vi "CTREPCM_PanelSim_Global.vi"(0 "Menu":T3=enum."delete", 5 "Channel":i32, 7 "Boolean Value":bool, 9 "Numeric Value":dbl format="%#.4f", 11 "error in (no error)":errorcluster, 12 "String Value":string) -> (10 "Value out":T1={"type"="CTREPCM", "device"="", "name"="", "data"={"<init"=FALSE, ">on"=FALSE, "<closed_loop"=FALSE, ">pressure_switch"=FALSE, ">current"=0.0}}, 15 "error out":errorcluster)   [LabVIEW 2019]
doc: "This is used to set and get the last motor output values. This is needed for simulation, since we cannot read these values from the hardware.\n\nThis software is licensed. Open the labview\\readme\\WPI Robotics Library Open Source License.txt file for more information."
uses:
  CTREPCM Update Ops.ctl
  CTREPCM proto.ctl
  CTREPCM Data proto.ctl
panel:
  out "All Values":T1[](array[typedef])
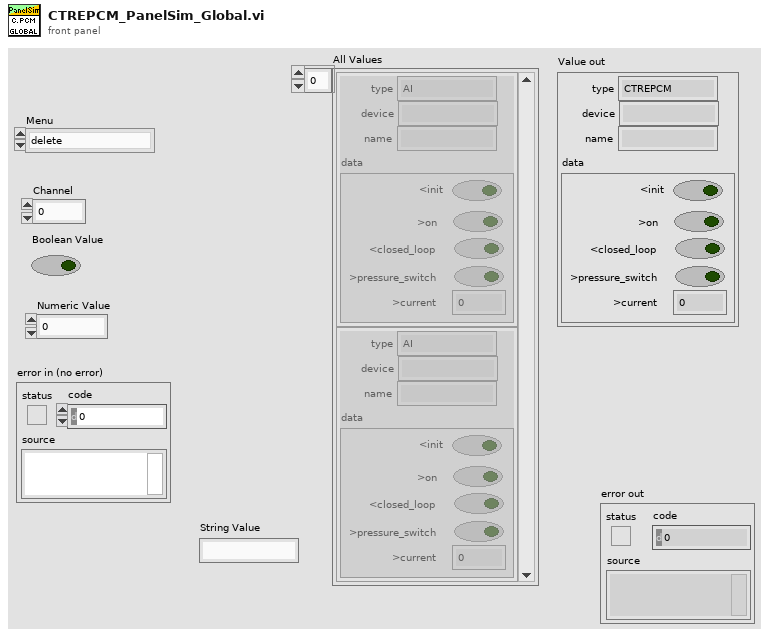
[diagram p1: front panel]
types:
  T1 = typedef "CTREPCM proto.ctl" = cluster{"type":string, "device":string, "name":string, "data":T2}
  T2 = typedef "CTREPCM Data proto.ctl" = cluster{"<init":bool, ">on":bool, "<closed_loop":bool, ">pressure_switch":bool, ">current":dbl}
  T3 = typedef "CTREPCM Update Ops.ctl" = enum16{"get", "delete", "JSON update", "set  name", "transmit initial", "reset", "set init", "set compressor on", "set closed loop", "set pressure switch", "set current"}
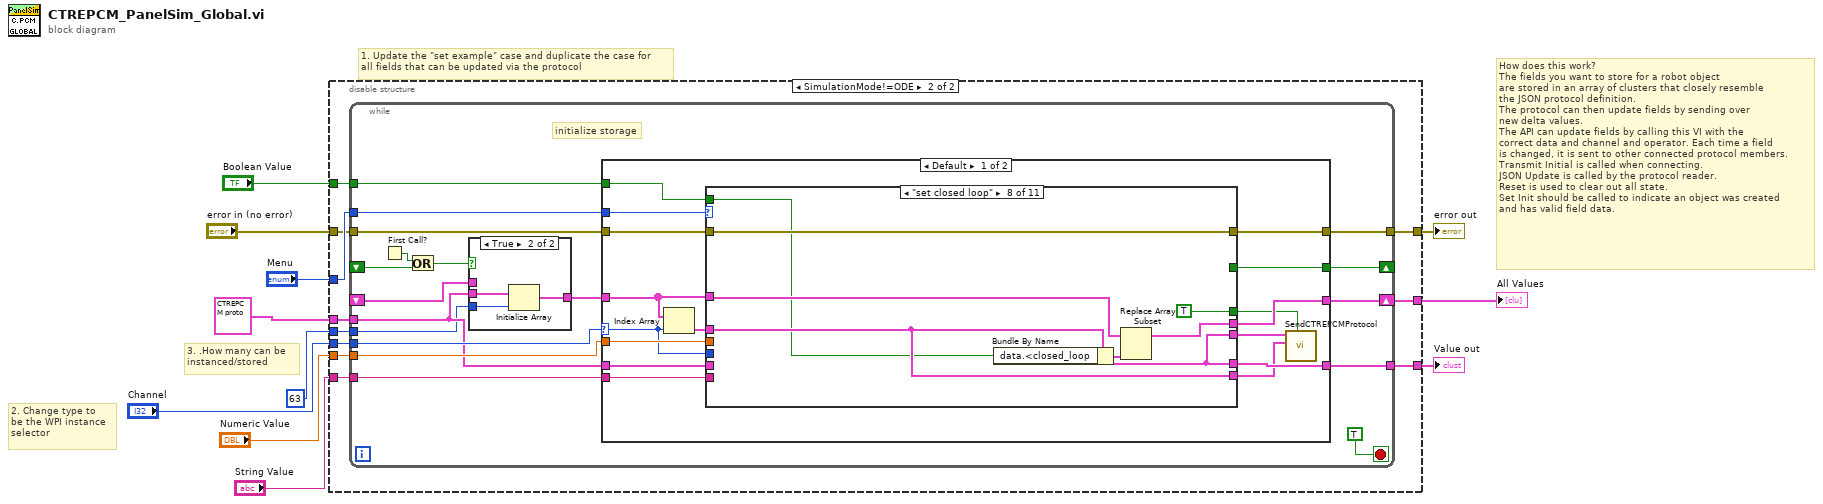
[diagram p0: block diagram]
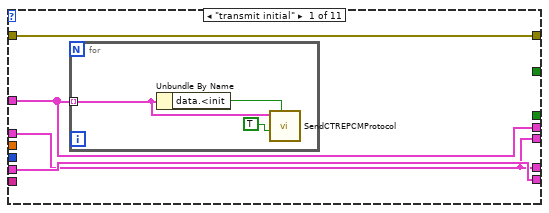
[diagram p3: hidden frame]
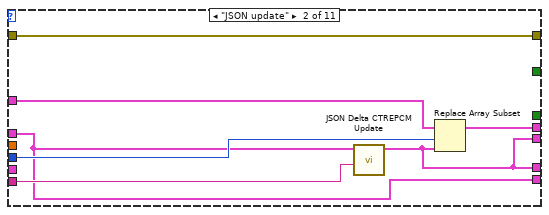
[diagram p4: hidden frame]
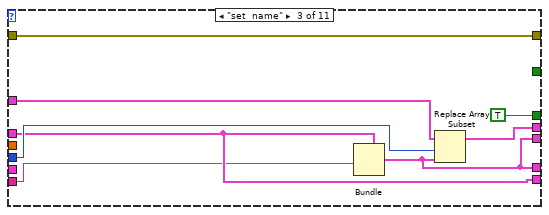
[diagram p5: hidden frame]
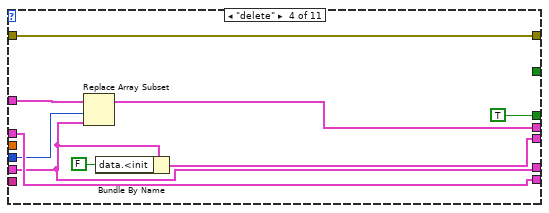
[diagram p6: hidden frame]
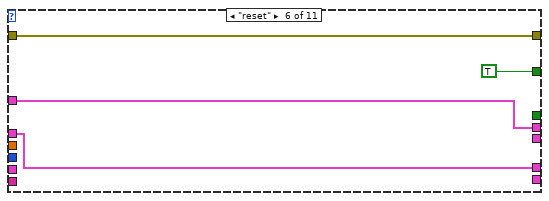
[diagram p8: hidden frame]
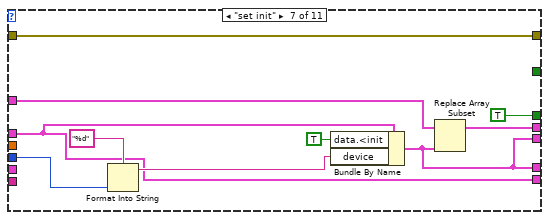
[diagram p9: hidden frame]
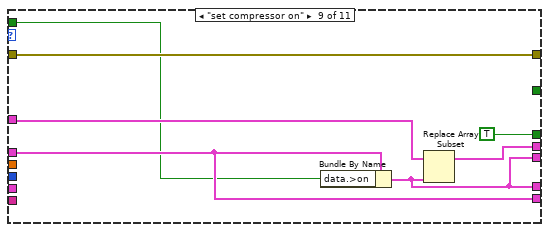
[diagram p10: hidden frame]
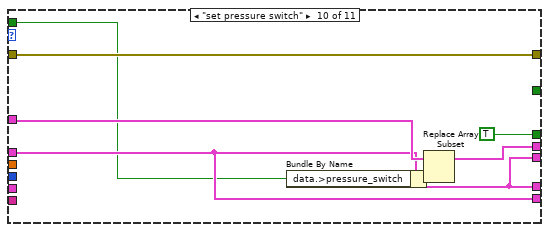
[diagram p11: hidden frame]
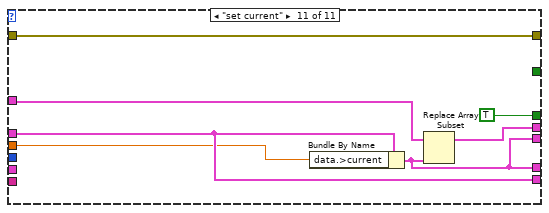
[diagram p12: hidden frame]
diagram:
  # "How does this work?\nThe fields you want to store for a robot object\nare stored in an array of clusters that closely resemble\nthe JSON protocol definition.\nThe protocol can then update fields by sending over\nnew delta values.\nThe API can update fields by calling this VI with the\ncorrect data and channel and operator. Each time a field\nis changed, it is sent to other connected protocol members.\nTransmit Initial is called when connecting.\nJSON Update is called by the protocol reader.\nReset is used to clear out all state.\nSet Init should be called to indicate an object was created\nand has valid field data."
  # "1. Update the \"set example\" case and duplicate the case for\nall fields that can be updated via the protocol"
  # "2. Change type to\nbe the WPI instance\nselector"
  # "3. .How many can be\ninstanced/stored"
  n1 = disable-structure shown="SimulationMode!=ODE" {
    disable-tunnel: "Menu" -> [_ w24]
    disable-tunnel: [w13 w23] -> w10
    disable-tunnel: "error in (no error)" -> [w13 w22]
    disable-tunnel: [_ w21] -> w8
    disable-tunnel: "Numeric Value" -> [_ w20]
    disable-tunnel: "Channel" -> [_ w19]
    disable-tunnel: [w12 w18] -> w5
    disable-tunnel: T1 {"type"="CTREPCM", "device"="", "name"="", "data"={"<init"=FALSE, ">on"=FALSE, "<closed_loop"=FALSE, ">pressure_switch"=FALSE, ">current"=0.0}} ("Accel value out") -> [w12 w17]
    disable-tunnel: "String Value" -> [_ w16]
    disable-tunnel: 63 -> [_ w15]
    disable-tunnel: "Boolean Value" -> [_ w14]
    frame condition #0 {
    }
    frame condition #1 (active) {
      n2 = while {
        tunnel: w20 -> [w42]
        tunnel: w22 -> [w38]
        shift-right: [w41] -> w21
        shift-left: _ -> [w34]
        tunnel: [w40] -> w18
        tunnel: w24 -> [w39]
        tunnel: [w37] -> w23
        tunnel: w19 -> [w33]
        tunnel: w17 -> [w32]
        tunnel: w16 -> [w31]
        shift-right: [w27] -> _
        shift-left: _ -> [w28]
        tunnel: w15 -> [w26]
        tunnel: w14 -> [w25]
        stop <- TRUE stop-if-true
        # "initialize storage"
        n3 = First Call?() -> (First Call?: T/F=w29:bool)
        n4 = Or(x=w29, y=w28) -> (x .or. y?=w30:bool)
        n5 = case shown="True" w30 {
          tunnel: [w138 w141] -> w35
          tunnel: w34 -> [w138 _]
          tunnel: w32 -> [_ w140]
          tunnel: w26 -> [_ w139]
          frame False {
          }
          frame True {
            n6 = Initialize Array(w140, w139) -> (w141:T1[])
          }
        }
        n7 = case shown="Default" w33 {
          selector: w33 -> [w51 _]
          tunnel: w42 -> [w58 _]
          tunnel: [w57 w137] -> w41
          tunnel: [w56 w135] -> w40
          tunnel: w39 -> [w55 _]
          tunnel: w38 -> [w54 w136]
          tunnel: [w53 w136] -> w37
          tunnel: w35 -> [w52 w137]
          tunnel: w32 -> [w49 w135]
          tunnel: w31 -> [w48 _]
          tunnel: [w47 _] -> w27
          tunnel: w25 -> [w43 _]
          frame Default {
            n8 = Index Array(array=w52, index=w51) -> (element=w50:T1)
            n9 = case shown="\"set closed loop\"" w55 {
              tunnel: w58 -> [_ _ _ _ _ _ _ _ _ _ w128]
              tunnel: [w59 w72 w80 w88 w92 w96 w102 w111 w118 w125 w132] -> w57
              tunnel: w52 -> [w59 w70 w78 w89 w92 w96 w101 w112 w119 w126 w133]
              tunnel: [w60 w68 w73 w82 w90 w94 w99 w108 w115 w122 w129] -> w56
              tunnel: [w62 w71 w79 w87 w91 w95 w98 w113 w120 w127 w134] -> w53
              tunnel: w54 -> [w62 w71 w79 w87 w91 w95 w98 w113 w120 w127 w134]
              tunnel: w51 -> [_ w69 w76 w84 _ _ w105 _ _ _ _]
              tunnel: [w60 w68 w73 w83 _ _ w99 w108 w115 w122 w129] -> w45
              tunnel: [w61 w66 w75 w85 _ _ w100 w109 w116 w123 w130] -> w44
              tunnel: [_ _ TRUE TRUE _ _ TRUE TRUE TRUE TRUE TRUE] -> w46
              tunnel: w50 -> [w60 w66 w75 w85 w90 w94 w100 w109 w116 w123 w130]
              tunnel: w49 -> [w61 _ _ w82 _ _ _ _ _ _ _]
              tunnel: w48 -> [_ w67 w74 _ _ _ _ _ _ _ _]
              tunnel: [_ _ _ _ _ TRUE _ _ _ _ _] -> w47
              tunnel: w43 -> [_ _ _ _ _ _ _ w107 w114 w121 _]
              frame "transmit initial" {
                n10 = for {
                  tunnel: w59 -> [w65] mode=indexing
                  n11 = Unbundle By Name(w65) -> ("data.<init"=w63:bool)
                  n12 = call "SendCTREPCMProtocol.vi"("Send"=w63, "Initialize"=TRUE ("Send"), "Current"=w65) -> ()  [unwired: 9 in]
                }
              }
              frame "JSON update" {
                n13 = call "JSON Delta CTREPCM Update.vi"("Delta JSON"=w67, "input"=w66) -> ("output"=w68:T1)  [unwired: 8 in, 1 out]
                n14 = Replace Array Subset(array=w70, new element=w68, index=w69) -> (w72:T1[])
              }
              frame "set  name" {
                n15 = Bundle(cluster=w75, "name"=w74) -> (w73:T1)  [unwired: 3 in]
                n16 = Replace Array Subset(array=w78, new element=w73, index=w76) -> (w80:T1[])
              }
              frame "delete" {
                n17 = Replace Array Subset(array=w89, new element=w82, index=w84) -> (w88:T1[])
                n18 = Bundle By Name(cluster=w82, "data.<init"=FALSE) -> (w83:T1)
              }
              frame "get" {
              }
              frame "reset" {
              }
              frame "set init" {
                n19 = Format Into String(format string="%d", w105) -> (resulting string=w104:string)  [unwired: 2 in, 1 out]
                n20 = Bundle By Name(cluster=w100, "data.<init"=TRUE, "device"=w104) -> (w99:T1)
                n21 = Replace Array Subset(array=w101, new element=w99) -> (w102:T1[])  [unwired: 1 in]
              }
              frame "set closed loop" {
                n22 = Bundle By Name(cluster=w109, "data.<closed_loop"=w107) -> (w108:T1)
                n23 = Replace Array Subset(array=w112, new element=w108) -> (w111:T1[])  [unwired: 1 in]
              }
              frame "set compressor on" {
                n24 = Bundle By Name(cluster=w116, "data.>on"=w114) -> (w115:T1)
                n25 = Replace Array Subset(array=w119, new element=w115) -> (w118:T1[])  [unwired: 1 in]
              }
              frame "set pressure switch" {
                n26 = Bundle By Name(cluster=w123, "data.>pressure_switch"=w121) -> (w122:T1)
                n27 = Replace Array Subset(array=w126, new element=w122) -> (w125:T1[])  [unwired: 1 in]
              }
              frame "set current" {
                n28 = Bundle By Name(cluster=w130, "data.>current"=w128) -> (w129:T1)
                n29 = Replace Array Subset(array=w133, new element=w129) -> (w132:T1[])  [unwired: 1 in]
              }
            }
            n30 = call "SendCTREPCMProtocol.vi"("Send"=w46, "Previous"=w44, "Current"=w45) -> ()  [unwired: 9 in]
          }
          frame -1 {
            # "Do nothing if \nchannel is Invalid."
          }
        }
      }
    }
  }
  "error out" <- w10
  "Value out" <- w5
  "All Values" <- w8
